vi "FlatToRichniswitch_grpc_RevisionQueryResponse.vi"(5 "OutputClusterType":T1, 11 "InputCluster":T2) -> (3 "OutputCluster":T1)   [LabVIEW 2021, in "NI Switch_client.lvlib"]
uses:
  NI Switch_client.lvlib
  niswitch_grpc_RevisionQueryResponse_Flat.ctl
  niswitch_grpc_RevisionQueryResponse.ctl
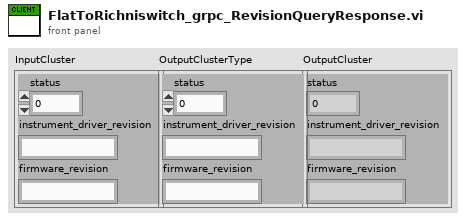
[diagram p1: front panel]
types:
  T1 = typedef "NI Switch_client.lvlib/niswitch_grpc_RevisionQueryResponse.ctl" = cluster{"status":i32, "instrument_driver_revision":string, "firmware_revision":string}
  T2 = typedef "NI Switch_client.lvlib/niswitch_grpc_RevisionQueryResponse_Flat.ctl" = cluster{"status":i32, "instrument_driver_revision":string, "firmware_revision":string}
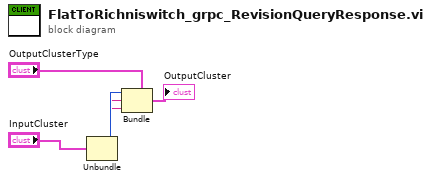
[diagram p0: block diagram]
diagram:
  n1 = Unbundle "Unbundle"("InputCluster") -> ("status"=w3:i32, "instrument_driver_revision"=w2:string, "firmware_revision"=w1:string)
  n2 = Bundle "Bundle"(cluster="OutputClusterType", "status"=w3, "instrument_driver_revision"=w2, "firmware_revision"=w1) -> (→"OutputCluster":T1)
